vi "AddtoTransfrom.vi"(8 "error in (no error)":errorcluster, 11 "TransformTokenizer in":refnum<class "TransformTokenizer.lvclass">) -> (0 "error out":errorcluster, 3 "TransformTokenizer out":refnum<class "TransformTokenizer.lvclass">)   [LabVIEW 2019, in "TransformTokenizer.lvclass"]
uses:
  TransformTokenizer.lvclass
  TransformTokenizer.lvclass/TransformTokenizer.ctl
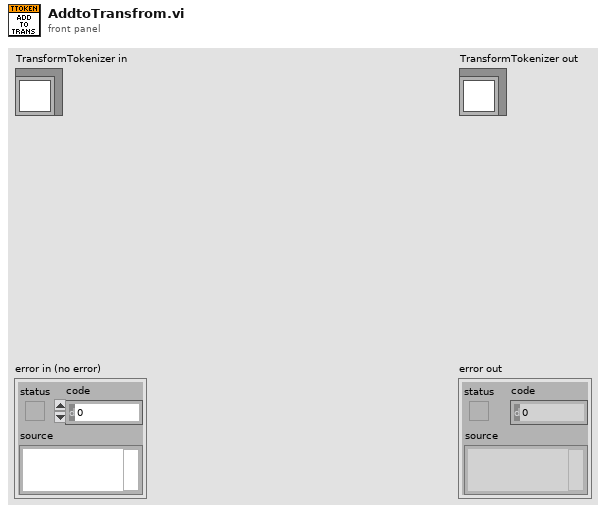
[diagram p1: front panel]
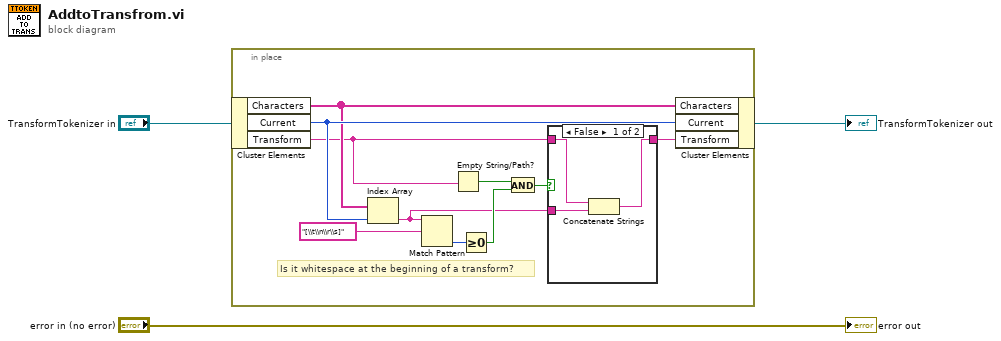
[diagram p0: block diagram]
diagram:
  n1 = in-place {
    # "Is it whitespace at the beginning of a transform?"
    n2 = in-place-cluster #1("TransformTokenizer in") -> ("Characters"=w12:string[], "Current"=w13:i32, "Transform"=w4:string)
    n3 = Index Array(array=w12, index=w13) -> (element=w5:string)
    n4 = Match Pattern(string=w5, regular expression="[\\t\\n\\r\\s]") -> (offset past match=w11:i32)  [unwired: 1 in, 3 out]
    n5 = Empty String/Path?(string/path=w4) -> (empty?=w9:bool)
    n6 = Greater Or Equal To 0?(x=w11) -> (x >= 0?=w10:bool)
    n7 = And(x=w9, y=w10) -> (x .and. y?=w8:bool)
    n8 = case shown="False" w8 {
      tunnel: w5 -> [w16 _]
      tunnel: [w15 w17] -> w7
      tunnel: w4 -> [w14 w17]
      frame False {
        n9 = Concatenate Strings(w14, w16) -> (w15:string)
      }
      frame True {
        # "If true dont add to transform"
      }
    }
    n10 = in-place-cluster #1("Characters"=w12, "Current"=w13, "Transform"=w7) -> (→"TransformTokenizer out":refnum<class "TransformTokenizer.lvclass">)
  }
  "error out" <- "error in (no error)"
